vi "Drag Start.vi"(8 "error in (no error)":errorcluster, 11 "BetterTreeHandle in":refnum<class "BetterTreeHandle.lvclass">) -> (0 "error out":errorcluster, 2 "BetterDropOp":refnum<class "BetterDropOp.lvclass">, 3 "BetterTreeHandle out":refnum<class "BetterTreeHandle.lvclass">)   [LabVIEW 2020, in "BetterDragAndDrop.lvlib" / "BetterTreeHandle.lvclass"]
uses:
  BetterTreeHandle.lvclass
  BetterDropOp/BetterDropOp.lvclass
  BetterTreeHandle.lvclass/BetterTreeHandle.ctl
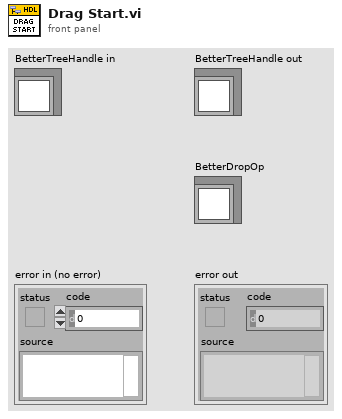
[diagram p1: front panel]
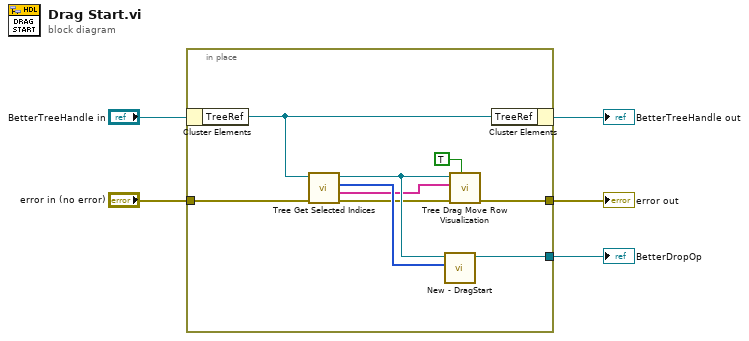
[diagram p0: block diagram]
diagram:
  n1 = in-place {
    in-place-border: "error in (no error)" -> [w12]
    in-place-border: [w7] -> w3
    in-place-border: [w6] -> w2
    n2 = in-place-cluster #1("BetterTreeHandle in") -> ("TreeRef"=w13:refnum<vi>)
    n3 = call "Tree Get Selected Indices.vi"("error in (no error)"=w12, "Tree Ref"=w13) -> ("error out"=w9:errorcluster, "Tree.Values"=w8:string[], "Selected Indices"=w11:i32[], "tree ref"=w10:refnum<vi>)  [unwired: 5 in, 1 out]
    n4 = call "New - DragStart.vi"("DragStart Indices"=w11, "Ref"=w10) -> ("BetterDropOp out"=w7:refnum<class "BetterDropOp.lvclass">)  [unwired: 8 in, 1 out]
    n5 = call "Tree Drag Move Row Visualization.vi"("DragStart? (F)"=TRUE ("Activate?"), "error in (no error)"=w9, "Active Item Tags"=w8, "TreeRef"=w10) -> ("error out"=w6:errorcluster)  [unwired: 7 in]
    n6 = in-place-cluster #1("TreeRef"=w13) -> (→"BetterTreeHandle out":refnum<class "BetterTreeHandle.lvclass">)
  }
  "error out" <- w2
  "BetterDropOp" <- w3
